vi "Bury.vi"(8 "Error In":errorcluster, 11 "Selection List[]":refnum<vi>[](array[refnum])) -> (0 "Error Out":errorcluster, 3 "Change Made?":bool)   [LabVIEW 2017, in "Toolkit.lvlib"]
doc: "Burys the corpse of legacy code. This removes the grave (Diagram Disable Structure) and leaves behind the Spirit frame, which should be enabled before burying the corpse. Note, the corpse frame will no longer exists and be pernamently deleted."
uses:
  Toolkit.lvlib
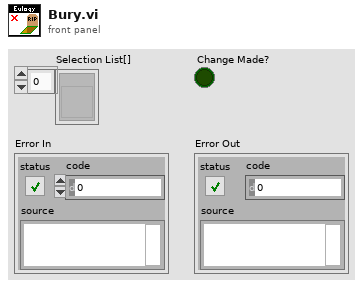
[diagram p1: front panel]
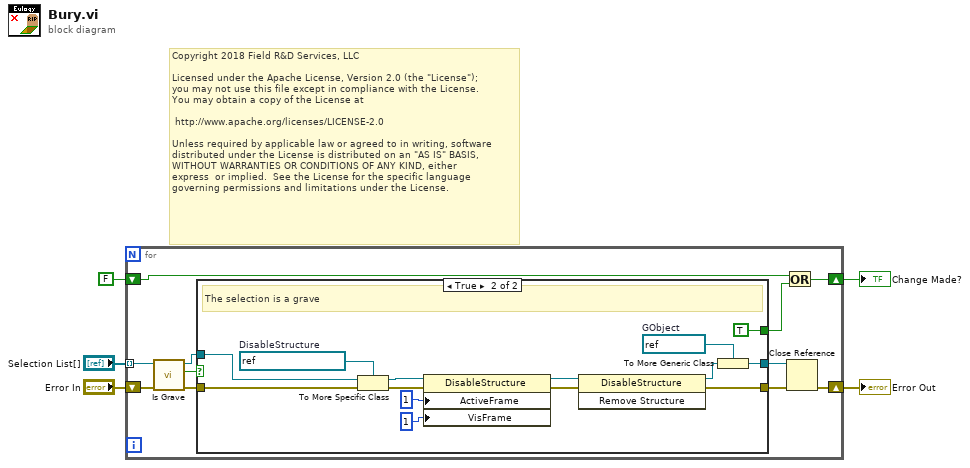
[diagram p0: block diagram]
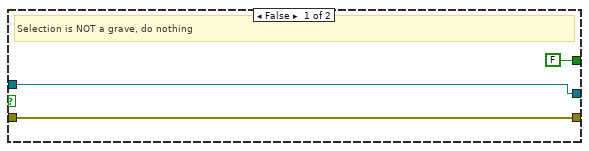
[diagram p2: hidden frame]
diagram:
  # "Copyright 2018 Field R&D Services, LLC\n\nLicensed under the Apache License, Version 2.0 (the \"License\");\nyou may not use this file except in compliance with the License.\nYou may obtain a copy of the License at\n\n\thttp://www.apache.org/licenses/LICENSE-2.0\n\nUnless required by applicable law or agreed to in writing, software\ndistributed under the License is distributed on an \"AS IS\" BASIS,\nWITHOUT WARRANTIES OR CONDITIONS OF ANY KIND, either \nexpress  or implied.  See the License for the specific language \ngoverning permissions and limitations under the License."
  n1 = for {
    shift-right: [w11] -> w5
    shift-left: "Error In" -> [w6]
    tunnel: "Selection List[]" -> [w10] mode=indexing
    shift-right: [w14] -> w3
    shift-left: FALSE -> [w16]
    n2 = call "Is Grave.vi"("Error In"=w6, "GObject In"=w10) -> ("Error Out"=w7:errorcluster, "Grave?"=w8:bool, "GObject Out"=w9:refnum<vi>)  [unwired: 7 in]
    n3 = case shown="True" w8 {
      tunnel: w9 -> [w18 w32]
      tunnel: w7 -> [w17 w31]
      tunnel: [FALSE ("y") TRUE ("y")] -> w15
      tunnel: [w17 w29] -> w13
      tunnel: [w18 w26] -> w12
      frame False {
        # "Selection is NOT a grave, do nothing"
      }
      frame True {
        w27 = refnum<vi> refnum  # GObject
        w33 = refnum<vi> refnum  # DisableStructure
        # "The selection is a grave"
        n4 = To More Specific Class(target class=w33, reference=w32, error in=w31) -> (specific class reference=w25:refnum<vi>, error out=w24:errorcluster)
        n5 = property class="DisableStructure"(reference=w25, error in=w24, "ActiveFrame"=i16 1 ("Active Frame"), "VisFrame"=u32 1 ("Visible Frame")) -> (reference out=w22:refnum<vi>, error out=w20:errorcluster)
        n6 = invoke class="DisableStructure" method="Remove Structure"(reference=w22, error in=w20) -> (reference out=w28:refnum<vi>, error out=w29:errorcluster)  [unwired: 1 in, 1 out]
        n7 = To More Generic Class(target class=w27, reference=w28) -> (generic class reference=w26:refnum<vi>)
      }
    }
    n8 = Or(x=w16, y=w15) -> (x .or. y?=w14:bool)
    n9 = Close Reference(reference=w12, error in (no error)=w13) -> (error out=w11:errorcluster)
  }
  "Error Out" <- w5
  "Change Made?" <- w3
